vi "Update Gage Plot.vi"(8 "error in (no error)":errorcluster, 10 "Data":dbl[](array[numeric]), 11 "Gage digitizer actor in":refnum<class "Gage digitizer actor.lvclass">) -> (0 "error out":errorcluster, 3 "Gage digitizer actor out":refnum<class "Gage digitizer actor.lvclass">)   [LabVIEW 2015, in "Gage digitizer actor.lvclass"]
uses:
  Gage digitizer actor.lvclass
  Gage digitizer actor.lvclass/Gage digitizer actor.ctl
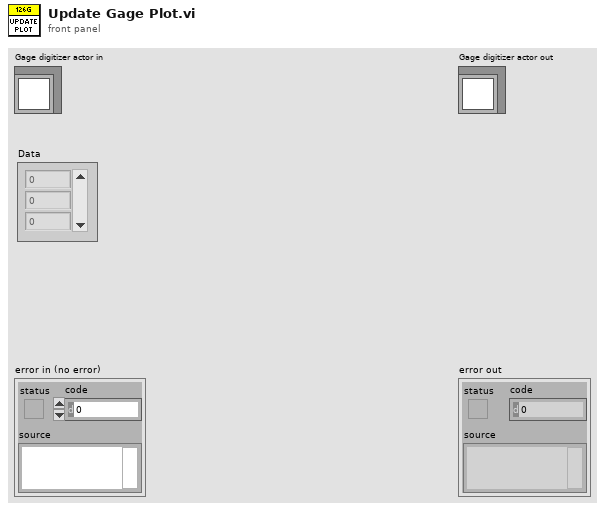
[diagram p1: front panel]
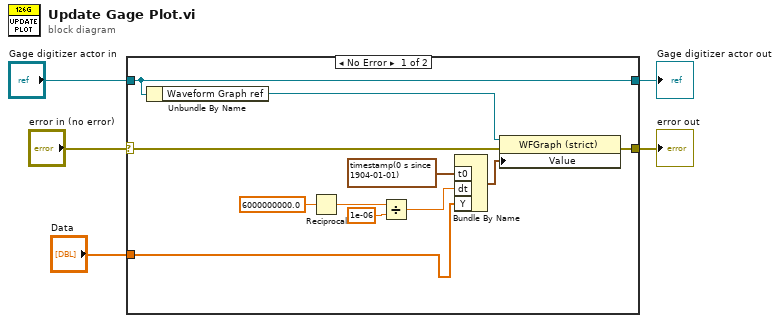
[diagram p0: block diagram]
diagram:
  n1 = case shown="No Error" "error in (no error)" {
    selector: "error in (no error)" -> [w8 w18]
    tunnel: [w9 w18] -> w4
    tunnel: [w16 w17] -> w2
    tunnel: "Gage digitizer actor in" -> [w16 w17]
    tunnel: "Data" -> [w6 _]
    frame No Error {
      n2 = Unbundle By Name(w16) -> ("Waveform Graph ref"=w10:refnum<vi>)
      n3 = Reciprocal(x=6000000000.0) -> (1/x=w15:dbl)
      n4 = Divide(x=w15, y=1e-06) -> (x/y=w12:dbl)
      n5 = Bundle By Name("t0"=timestamp(0 s since 1904-01-01), "dt"=w12, "Y"=w6) -> (w11:waveform(dbl))  [unwired: 1 in]
      n6 = property class="WFGraph (strict)"(reference=w10, error in=w8, "Value"=w11) -> (error out=w9:errorcluster)  [unwired: 1 out]
    }
    frame Error {
    }
  }
  "error out" <- w4
  "Gage digitizer actor out" <- w2
